vi "Limelight Basic Target Tracking.vi"() -> ()   [LabVIEW 2020]
uses:
  <vilib>/Rock Robotics/Network Tables/NT Read Number.vi
  <vilib>/Rock Robotics/WPI/Utilities/WPI_GetSetVariantRefNum.vi
  <vilib>/Rock Robotics/WPI/RobotDrive/WPI_RobotDriveArcadeDrive_Standard(NoSaturation).vi
panel:
  in  "Joystick Y - Throtle":dbl
  out "TX":dbl
  in  "Joystick X - Wheel":dbl
  in  "BUT 10":bool
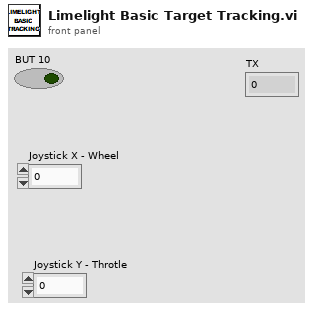
[diagram p1: front panel]
types:
  T1 = typedef "WPI_RobotDriveDevRef.ctl" = cluster{"DevStatus":errorcluster, "Motors[]":T2[], "Square Inputs":bool, "Max Output":dbl}
  T2 = typedef "WPI_MotorControlDeviceRef.ctl" = cluster{"DeviceStatus":errorcluster, "Type":T3, "PWM":cluster{"PWM Channel":T4, "DeadBand":T5}, "CAN":cluster{"Device Number":u8, "SetOutput VI Ref":variant, "GetOutput VI Ref":variant, "Enable VI Ref":variant, "Disable VI Ref":variant, "Data":variant}, "Invert":bool, "DIO PWM":cluster{"PWM \"Enable\" Channel":T4, "DIOChannel":T6, "PWM Rate":dbl}}
  T3 = typedef "WPI_MotorControlType.ctl" = enum16{"PWM", "CAN", "DIO PWM"}
  T4 = typedef "FPGA_DIOPWMChannel.ctl" = enum8{"PWM 0", "PWM 1", "PWM 2", "PWM 3", "PWM 4", "PWM 5", "PWM 6", "PWM 7", "PWM 8", "PWM 9", "PWM MXP 0", "PWM MXP 1", "PWM MXP 2", "PWM MXP 3", "PWM MXP 4", "PWM MXP 5", "PWM MXP 6", "PWM MXP 7", "PWM MXP 8", "PWM MXP 9", "Invalid"}
  T5 = typedef "WPI_PWMDeadband.ctl" = cluster{"Name":string, "maxPositivePwm":i32, "minPositivePwm":i32, "centerPwm":i32, "maxNegativePwm":i32, "minNegativePwm":i32, "angularRange":u16}
  T6 = typedef "FPGA_DIOChannel.ctl" = enum8{"DIO 0", "DIO 1", "DIO 2", "DIO 3", "DIO 4", "DIO 5", "DIO 6", "DIO 7", "DIO 8", "DIO 9", "DIO MXP 0", "DIO MXP 1", "DIO MXP 2", "DIO MXP 3", "DIO MXP 4", "DIO MXP 5", "DIO MXP 6", "DIO MXP 7", "DIO MXP 8", "DIO MXP 9", "DIO MXP 10", "DIO MXP 11", "DIO MXP 12", "DIO MXP 13", "DIO MXP 14", "DIO MXP 15", "SPI Port CS1", "SPI Port CS2", "SPI Port CS3", "SPI Port MISO", "SPI Port MOSI", "Invalid"}
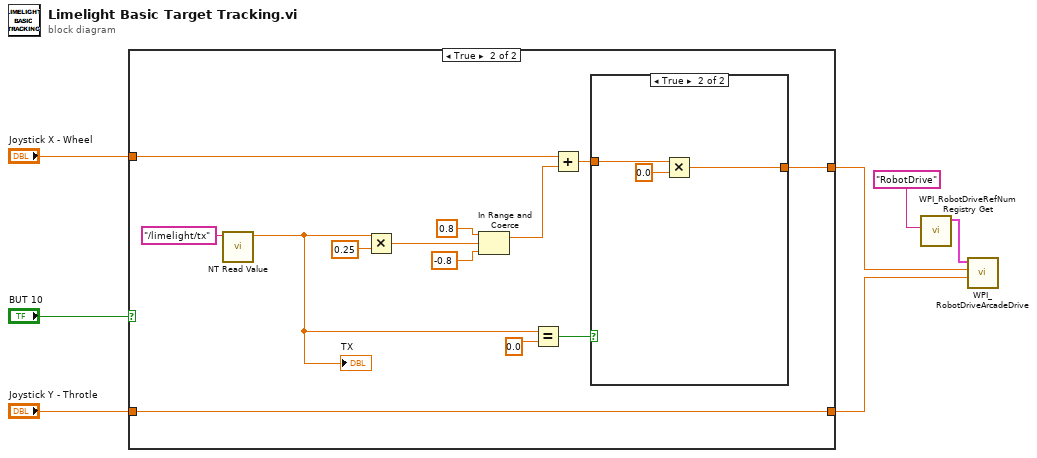
[diagram p0: block diagram]
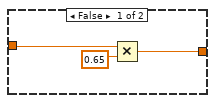
[diagram p3: hidden frame]
diagram:
  n1 = case shown="True" "BUT 10" {
    tunnel: [w9 w15] -> w7
    tunnel: [w8 w11] -> w6
    tunnel: "Joystick X - Wheel" -> [w9 w12]
    tunnel: "Joystick Y - Throtle" -> [w8 w11]
    frame False {
    }
    frame True {
      n2 = call-poly <vilib>:"NT Read Value.vi"("Name"="/limelight/tx") -> ("Numeric"=w10:dbl)  [unwired: 9 in, 1 out]
      "TX" <- w10
      n3 = Multiply(x=w10, y=0.25) -> (x*y=w20:dbl)
      n4 = In Range and Coerce(upper limit=0.8, x=w20, lower limit=-0.8) -> (coerced(x)=w21:dbl)  [unwired: 1 out]
      n5 = Equal?(x=w10, y=0.0) -> (x = y?=w14:bool)
      n6 = Add(x=w12, y=w21) -> (x+y=w16:dbl)
      n7 = case shown="True" w14 {
        tunnel: w16 -> [w24 w28]
        tunnel: [w25 w26] -> w15
        frame False {
          n8 = Multiply(x=w24, y=0.65) -> (x*y=w25:dbl)
        }
        frame True {
          n9 = Multiply(x=w28, y=0.0) -> (x*y=w26:dbl)
        }
      }
    }
  }
  n10 = call <vilib>:"WPI_RobotDriveRefNum Registry Get.vi"("refnum name"="RobotDrive") -> ("RobotDriveDevRef"=w2:T1)  [unwired: 9 in, 1 out]
  n11 = call-poly <vilib>:"WPI_RobotDriveArcadeDrive.vi"("Y axis value"=w6, "X axis value"=w7, "RobotDriveDevRef"=w2) -> ()  [unwired: 6 in, 3 out]
